vi "Start.vi"(8 "error in (no error)":errorcluster, 11 "Electrophysiology in":refnum<class "BehaviorData.lvclass">) -> (0 "error out":errorcluster, 3 "Electrophysiology out":refnum<class "BehaviorData.lvclass">)   [LabVIEW 2010, in "BehaviorData.lvclass"]
uses:
  BehaviorData.lvclass
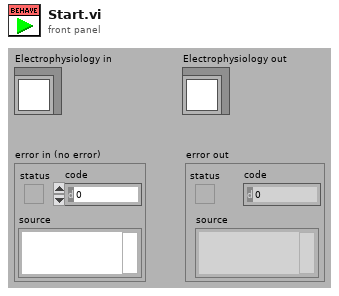
[diagram p1: front panel]
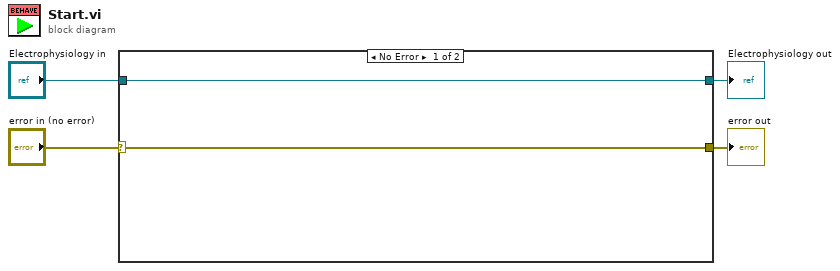
[diagram p0: block diagram]
diagram:
  n1 = case shown="No Error" "error in (no error)" {
    selector: "error in (no error)" -> [w5 w8]
    tunnel: [w5 w8] -> w3
    tunnel: [w6 w7] -> w1
    tunnel: "Electrophysiology in" -> [w6 w7]
    frame No Error {
    }
    frame Error {
    }
  }
  "error out" <- w3
  "Electrophysiology out" <- w1
